vi "File.Copy Source Dir to Targert Dir, Only Newer Files.vi"(10 "Target Dir":path, 11 "Source Dir":path) -> (0 "Error Out":errorcluster, 3 "Copied Files":path[](array[path]))   [LabVIEW 2018]
uses:
  <vilib>/KATE/Files/File Utils.lvlib
panel:
  in  "error in (no error)":errorcluster
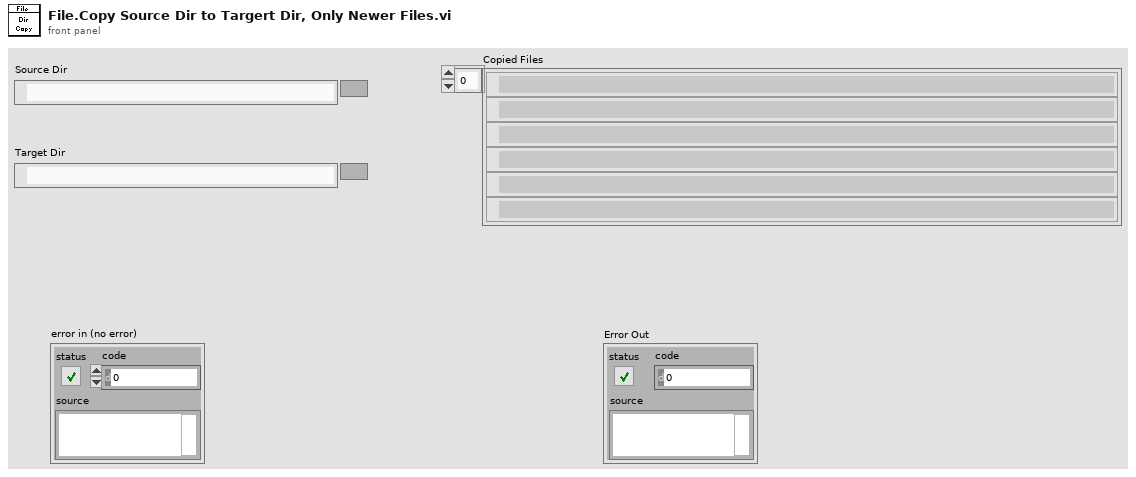
[diagram p1: front panel]
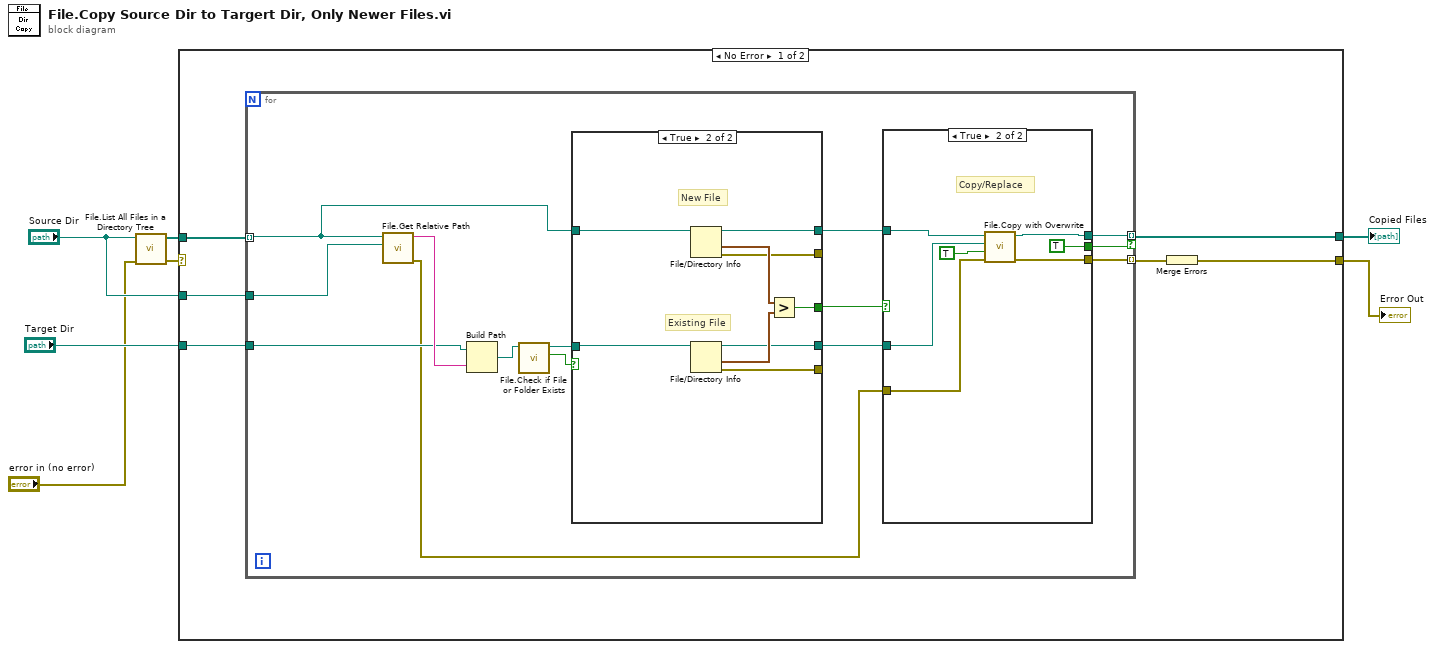
[diagram p0: block diagram]
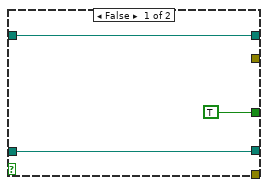
[diagram p3: hidden frame]
diagram:
  n1 = call <vilib>:"File.List All Files in a Directory Tree.vi"("error in (no error)"="error in (no error)", "Folder"="Source Dir") -> ("error out"=w4:errorcluster, "Files"=w7:path[])  [unwired: 8 in]
  n2 = case shown="No Error" w4 {
    selector: w4 -> [_ w47]
    tunnel: w7 -> [w13 _]
    tunnel: "Source Dir" -> [w12 _]
    tunnel: "Target Dir" -> [w11 _]
    tunnel: [w9 w47] -> w2
    tunnel: [w8 _] -> w3
    frame No Error {
      n3 = for {
        tunnel: w13 -> [w24] mode=indexing
        tunnel: w12 -> [w27]
        tunnel: w11 -> [w25]
        tunnel: [w17] -> w10 mode=indexing
        tunnel: [w16] -> w8 mode=indexing if=w15
        n4 = call "File.Get Relative Path.vi"("Root Dir"=w27, "Path"=w24) -> ("error out"=w14:errorcluster, "Relative Path"=w26:string)  [unwired: 8 in]
        n5 = Build Path(base path=w25, name or relative path=w26) -> (appended path=w23:path)
        n6 = call <vilib>:"File.Check if File or Folder Exists.vi"("Path"=w23) -> ("Exists"=w21:bool, "Dup Path"=w22:path)  [unwired: 6 in, 3 out]
        n7 = case shown="True" w21 {
          tunnel: w24 -> [w36 w46]
          tunnel: w22 -> [w35 w45]
          tunnel: [TRUE w42] -> w20
          tunnel: [w36 w41] -> w19
          tunnel: [w35 w40] -> w18
          tunnel: [_ w39] -> _
          tunnel: [_ w38] -> _
          frame False {
          }
          frame True {
            # "Existing File"
            # "New File"
            n8 = File/Directory Info(path=w46) -> (path out=w41:path, last mod=w44:timestamp, error out=w38:errorcluster)  [unwired: 1 in, 4 out]
            n9 = File/Directory Info(path=w45) -> (path out=w40:path, last mod=w43:timestamp, error out=w39:errorcluster)  [unwired: 1 in, 4 out]
            n10 = Greater?(x=w44, y=w43) -> (0:w42:bool)
          }
        }
        n11 = case shown="True" w20 {
          tunnel: w19 -> [_ w34]
          tunnel: w18 -> [_ w33]
          tunnel: [_ w32] -> w17
          tunnel: [_ w30] -> w16
          tunnel: [_ TRUE] -> w15
          tunnel: w14 -> [_ w29]
          frame False {
            # "Ignore"
          }
          frame True {
            # "Copy/Replace"
            n12 = call <vilib>:"File.Copy with Overwrite.vi"("error in (no error)"=w29, "Dest is Dir(F)/File(T)"=TRUE, "Destination"=w33, "Source"=w34) -> ("error out"=w32:errorcluster, "Destination Dup"=w30:path)  [unwired: 5 in, 1 out]
          }
        }
      }
      n13 = Merge Errors(w10) -> (w9:errorcluster)
    }
    frame Error {
    }
  }
  "Copied Files" <- w3
  "Error Out" <- w2
